vi "Read Module Menu Name.vi"(8 "error in":errorcluster, 11 "Logic Sequencer editor node in":refnum<class "Logic Sequencer editor node.lvclass">) -> (0 "error out":errorcluster, 2 "Menu Name":string, 3 "Logic Sequencer editor node out":refnum<class "Logic Sequencer editor node.lvclass">)   [LabVIEW 2013, in "Logic Sequencer editor node.lvclass"]
uses:
  Logic Sequencer editor node.lvclass
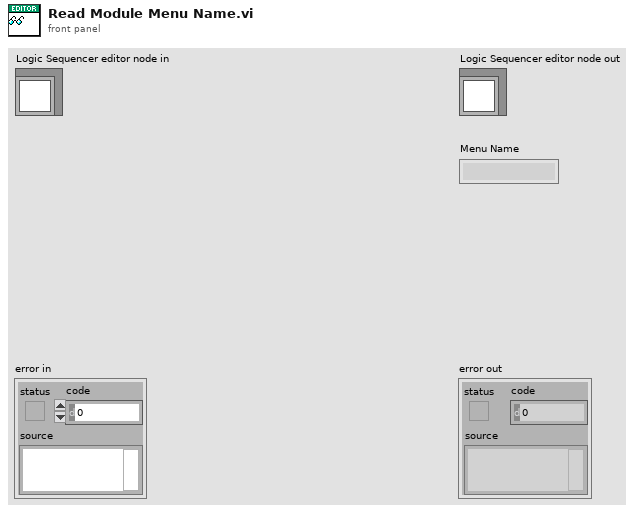
[diagram p1: front panel]
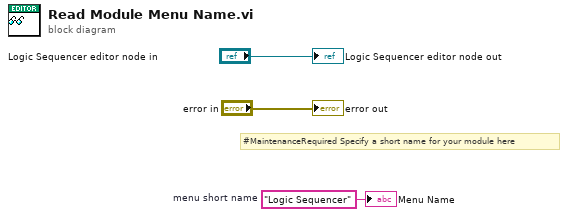
[diagram p0: block diagram]
diagram:
  w1 = "Logic Sequencer"  # menu short name
  # "#MaintenanceRequired Specify a short name for your module here"
  "error out" <- "error in"
  "Logic Sequencer editor node out" <- "Logic Sequencer editor node in"
  "Menu Name" <- w1
